vi "S2 Tool Initial.vi"(10 "process cluster":cluster{string[], i32[]}, 11 "Step Content":string[][](array[string])) -> (0 "error constant":errorcluster, 3 "S2 Initial Status":bool)   [LabVIEW 2019]
uses:
  Ctrl/StationCmdSelect.ctl
  Ctrl/Auto Inspection Station Name2.ctl
  Ctrl/Auto Inspection Data Name.ctl
  Global/Process Global.vi
  LineScan.lvclass
panel:
  in  "error in (no error)":errorcluster
  out "ToolStringOut_Init":string
  out "Initial_ChkSum":string
  in  "Numeric 3":i32
  out "Act Step":i32
  out "Numeric":dbl
  out "subarray":string[](array[string])
  out "Initial receive":string
  in  "stop":bool
  out "retry次數":string[](array[string])
  out "CurrentCmd":string
  out "Retry":i32
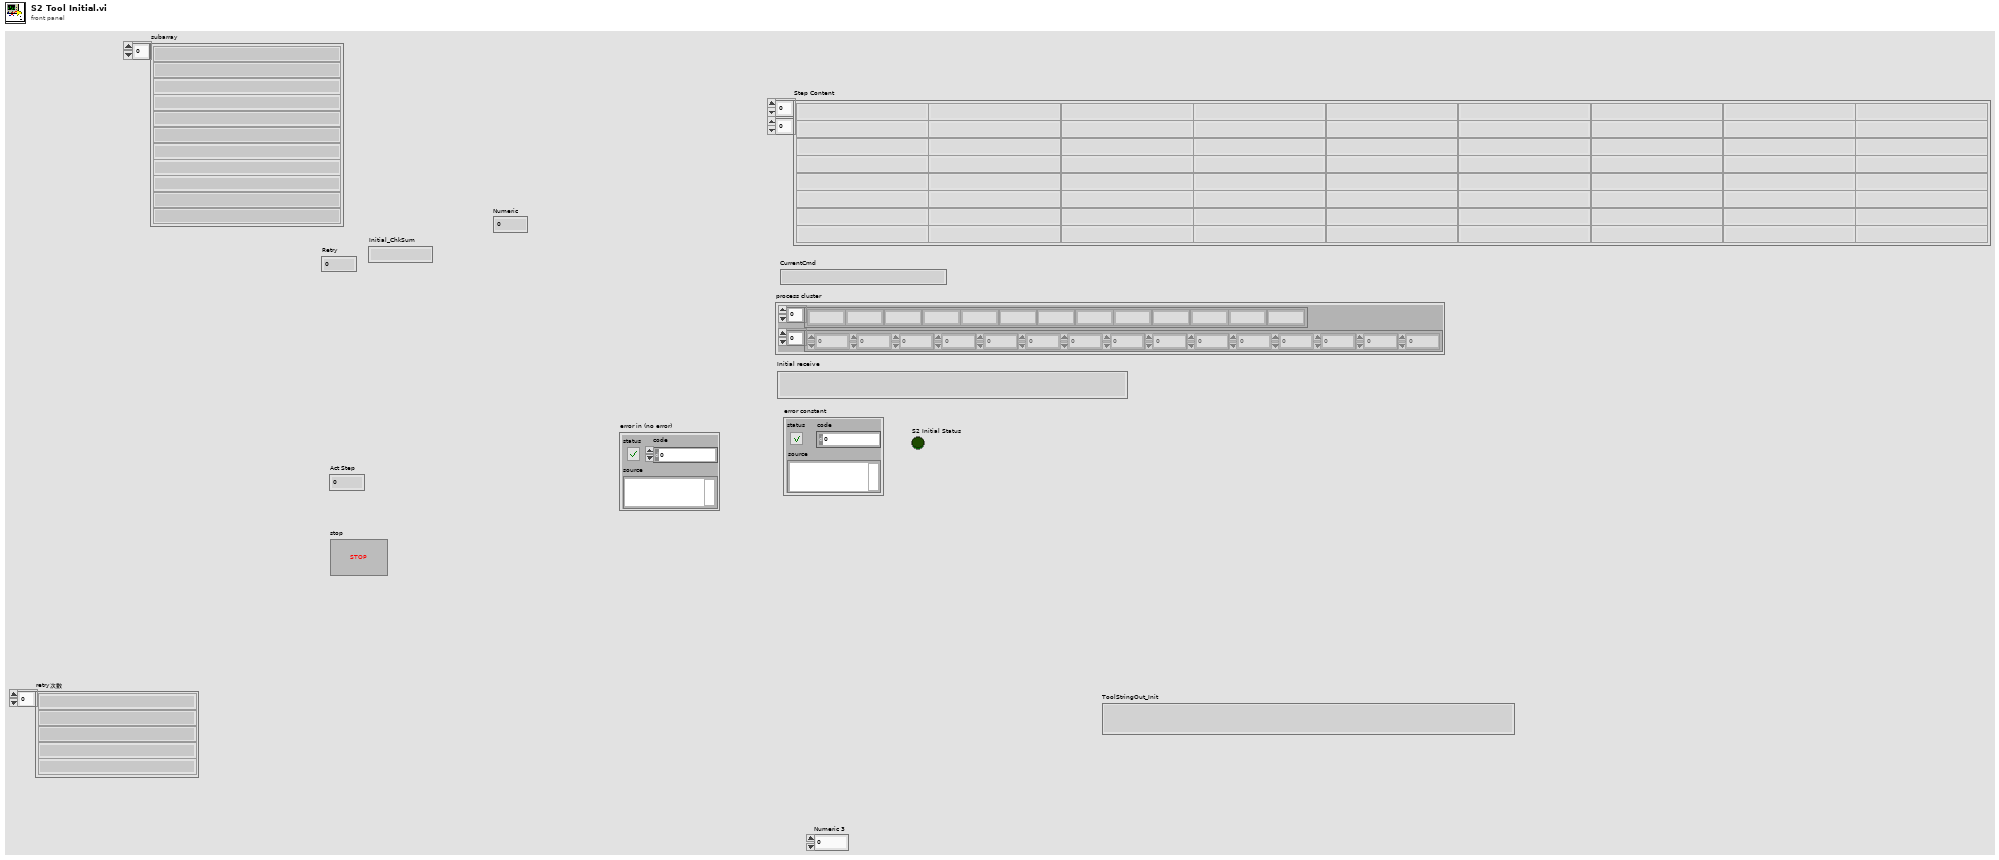
[diagram p1: front panel]
types:
  T1 = typedef "StationCmdSelect.ctl" = enum16{"Action", "Command", "Return", "DTime", "Retry"}
  T2 = typedef "Auto Inspection Data Name.ctl" = enum16{"LocalRun", "ItemSN(TimeCode)", "CurrentAction", "Error", "Data", "OKNG", "電壓值", "電壓值判斷", "電流值", "電流值判斷", "Laser1 Data", "Laser2 Data", "Laser OKNG", "StationNO"}
  T3 = typedef "Auto Inspection Station Name2.ctl" = enum16{"S1Barcode", "S2Measure", "S3Measure", "S4Measure", "S5Measure", "S11_LaserCheck", "S8_Vision AI"}
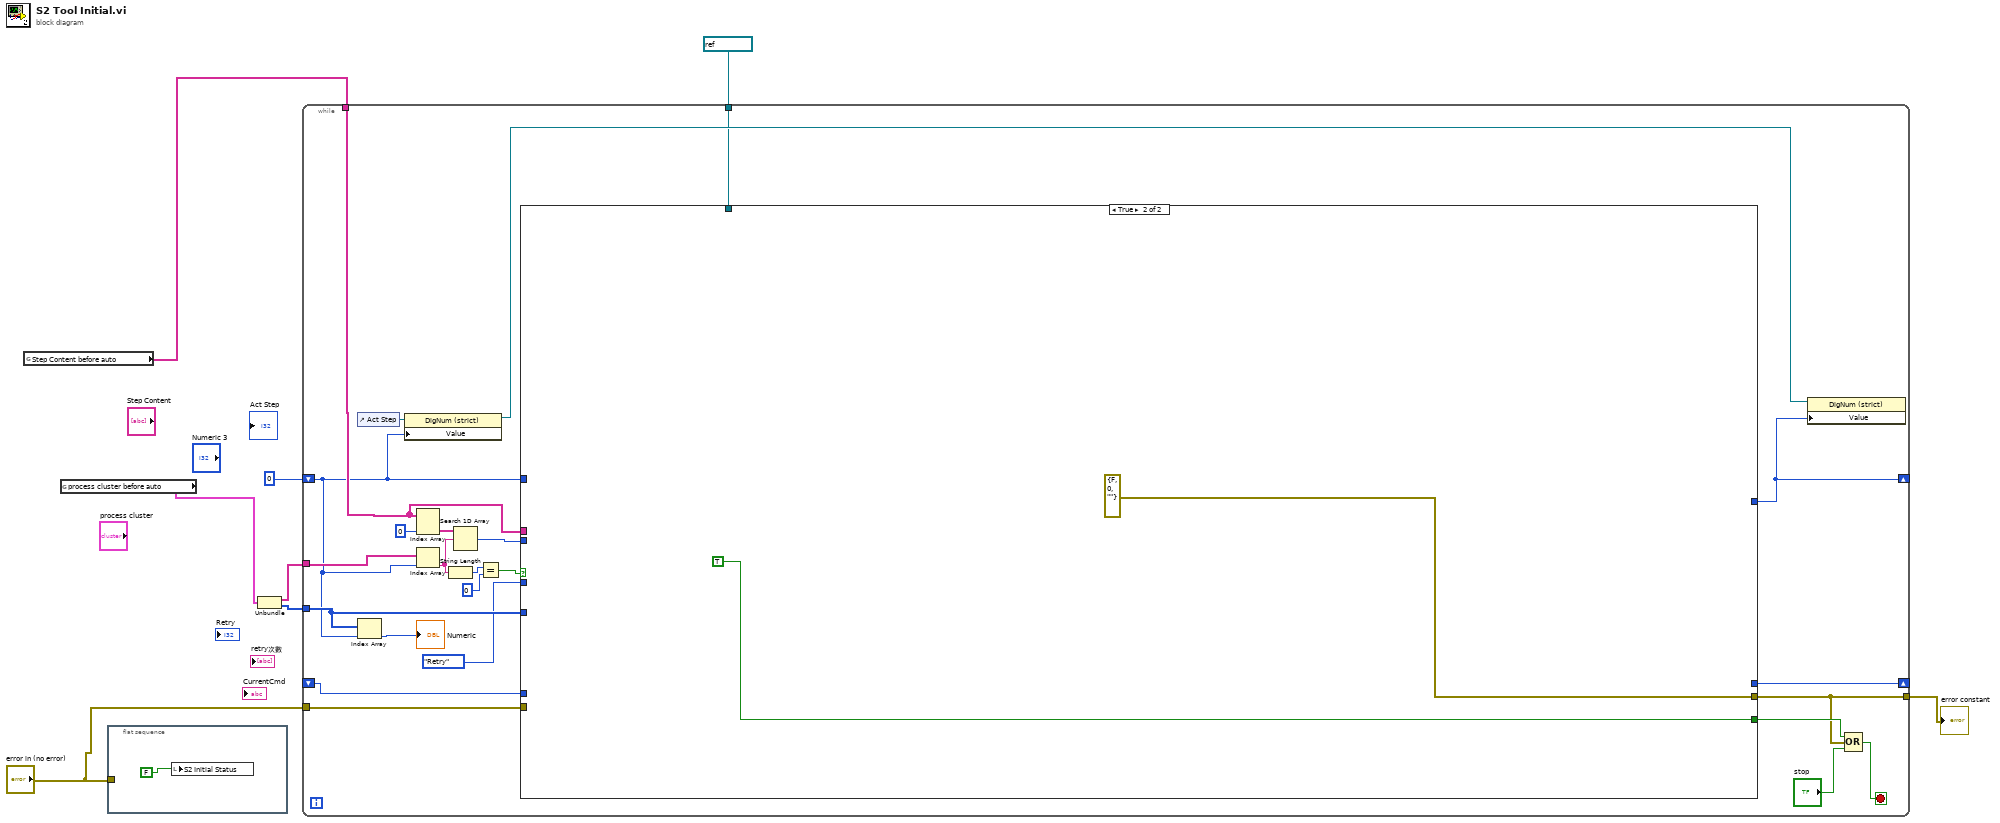
[diagram p0: block diagram]
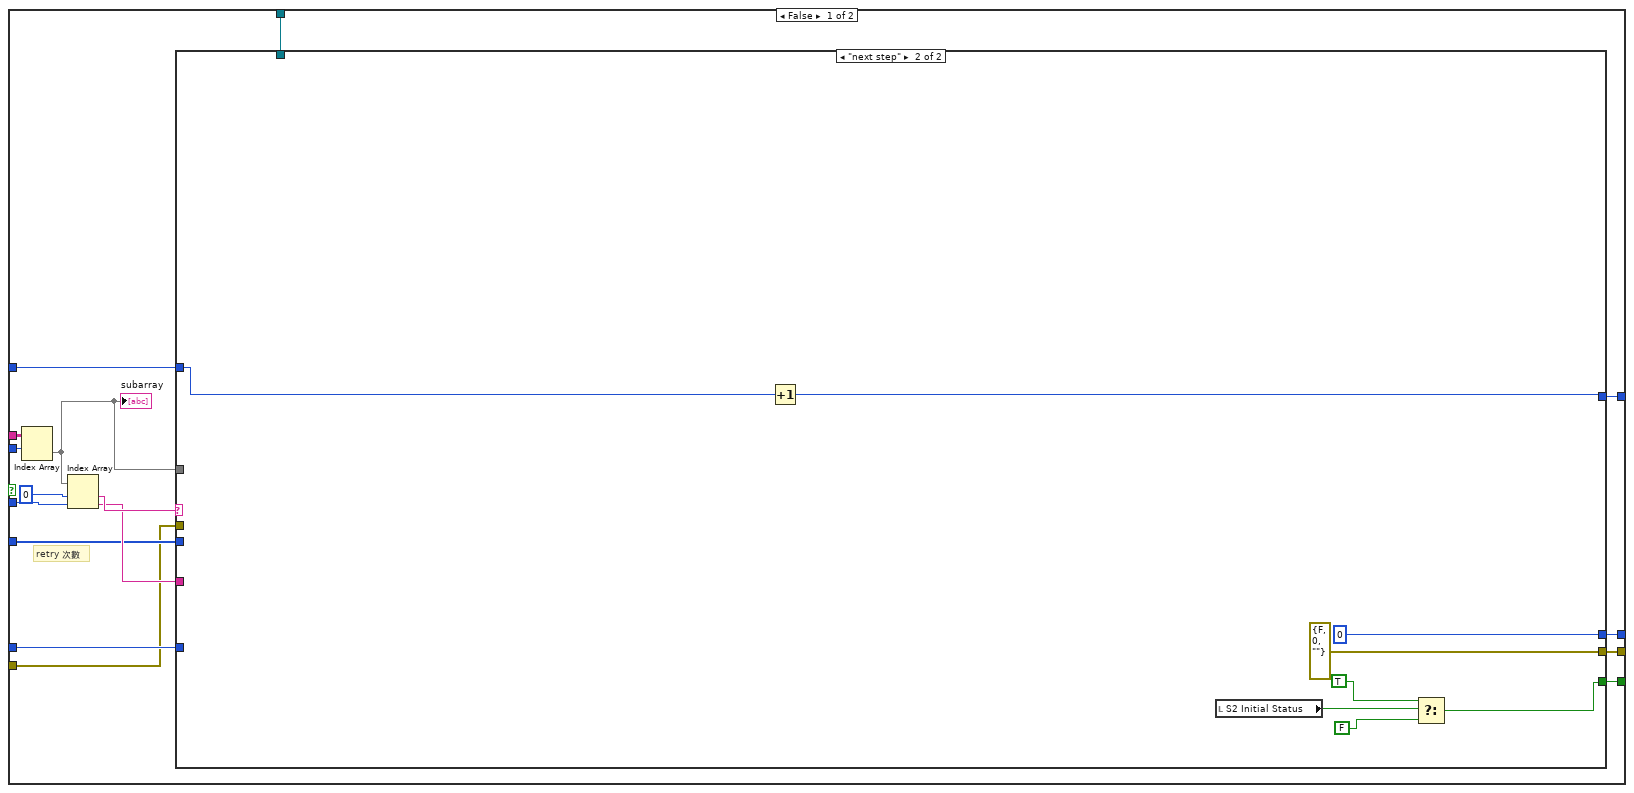
[diagram p2: hidden frame]
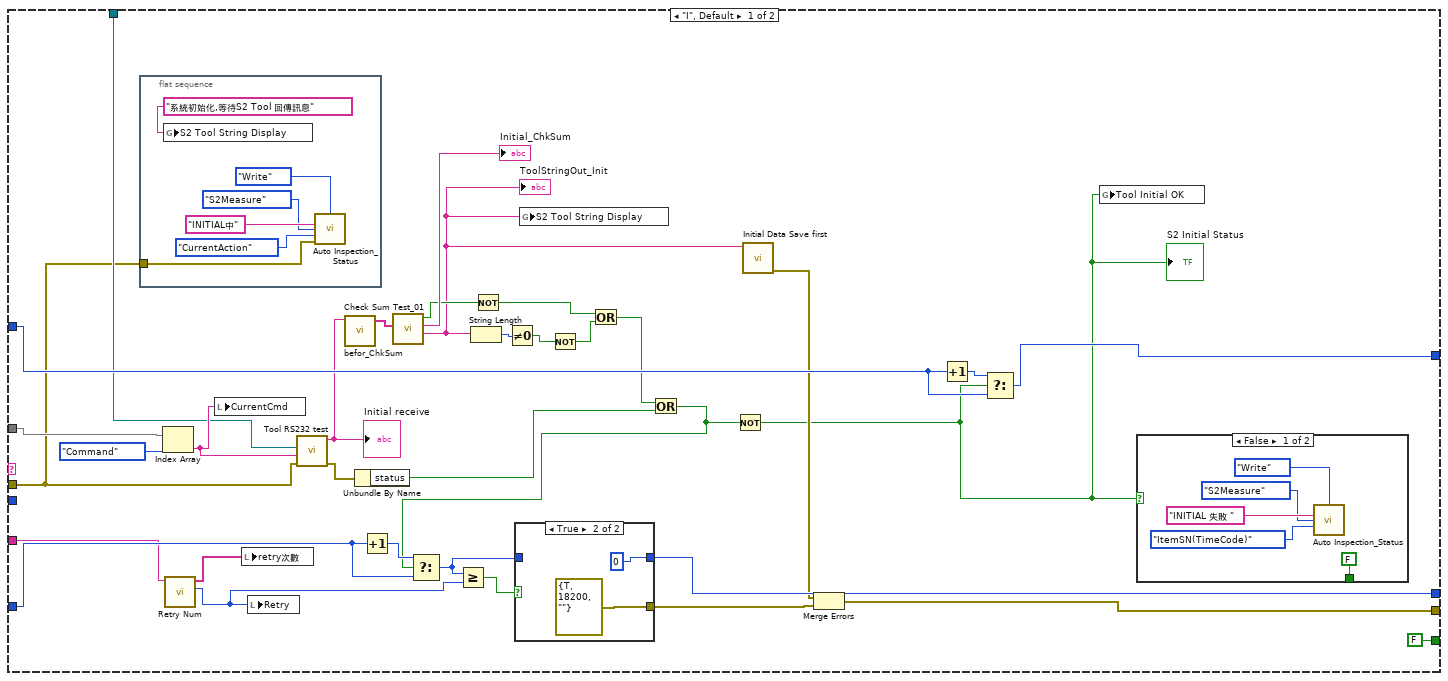
[diagram p3: hidden frame]
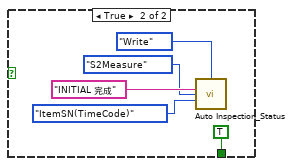
[diagram p4: hidden frame]
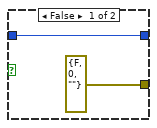
[diagram p5: hidden frame]
diagram:
  n1 = global read "Process Global.vi" "Step Content before auto"() -> (w5:string[][])
  n2 = global read "Process Global.vi" "process cluster before auto"() -> (w4:cluster{string[], i32[]})
  n3 = flat-sequence {
    tunnel: "error in (no error)" -> [_]
    frame #0 {
      n4 = local write "S2 Initial Status"(FALSE) -> ()
    }
  }
  n5 = Unbundle(w4) -> (w8:string[], w7:i32[])
  n6 = while {
    tunnel: w8 -> [w33]
    tunnel: w7 -> [w32]
    tunnel: w5 -> [w31]
    shift-right: [w15] -> _
    shift-left: _ -> [w19]
    shift-right: [w16] -> _
    shift-left: 0 ("Numeric 3") -> [w13]
    tunnel: [w12] -> w6
    tunnel: refnum<visa-resource-name> "COM1" ("VISA resource name") -> [w11]
    tunnel: "error in (no error)" -> [w10]
    stop <- w20 stop-if-true
    n7 = control-ref of="Act Step"() -> (w18:refnum<vi>)
    n8 = Index Array(array=w32, index=w13) -> (element=→"Numeric":i32)
    n9 = property class="DigNum (strict)"(reference=w18, "Value"=w13) -> (reference out=w17:refnum<vi>)  [unwired: 1 in, 1 out]
    n10 = Index Array(array=w31, index (col)=0 ("disabled index (col)")) -> (element=w29:string[])  [unwired: 1 in]
    n11 = Index Array(array=w33, index=w13) -> (element=w26:string)
    n12 = String Length(string=w26) -> (length=w25:i32)
    n13 = Search 1D Array(1D array=w29, element=w26) -> (index of element=w28:i32)  [unwired: 1 in]
    n14 = Equal?(x=w25, y=0) -> (x = y?=w23:bool)
    n15 = case shown="True" w23 {
      tunnel: w31 -> [w49 _]
      tunnel: w28 -> [w48 _]
      tunnel: w32 -> [w44 _]
      tunnel: w19 -> [w42 _]
      tunnel: StationCmdSelect."Retry" -> [w41 _]
      tunnel: [w40 errorcluster {"status"=FALSE, "code"=0, "source"=""} ("error constant")] -> w12
      tunnel: w13 -> [w39 _]
      tunnel: [w38 _] -> w16
      tunnel: [w37 _] -> w15
      tunnel: [w36 TRUE] -> w14
      tunnel: w11 -> [w35 _]
      tunnel: w10 -> [w34 _]
      frame False {
        # "retry 次數"
        n16 = Index Array(array=w49, index (row)=w48) -> (element=w43:string[])  [unwired: 1 in]
        "subarray" <- w43
        n17 = Index Array(array=w43, index #1=0 ("index"), index #2=w41) -> (element #1=w46:string, element #2=w45:string)
        n18 = case shown="\"next step\"" w46 {
          tunnel: w44 -> [_ _]
          tunnel: w45 -> [w72 _]
          tunnel: w43 -> [w74 _]
          tunnel: w42 -> [w73 _]
          tunnel: [w57 errorcluster {"status"=FALSE, "code"=0, "source"=""} ("error constant")] -> w40
          tunnel: w39 -> [w75 w111]
          tunnel: [w71 w110] -> w38
          tunnel: [w76 0] -> w37
          tunnel: [FALSE w104] -> w36
          tunnel: w34 -> [w51 _]
          tunnel: w35 -> [w56 _]
          frame "I", Default {
            n19 = flat-sequence {
              tunnel: w51 -> [w85]
              frame #0 {
                n20 = global write "Process Global.vi" "S2 Tool String Display"("系統初始化,等待S2 Tool 回傳訊息") -> ()
                n21 = call "Auto Inspection_Status.vi"("Action"=enum16{"Initial", "Write", "Read"}."Write", "DataIn"="INITIAL中", "Station"=Auto_Inspection_Station_Name2."S2Measure", "Data"=Auto_Inspection_Data_Name."CurrentAction", "error in"=w85) -> ()  [unwired: 8 in, 3 out]
              }
            }
            n22 = Index Array(array=w74, index=StationCmdSelect."Command") -> (element=w61:string)
            n23 = call "Retry Num.vi"("String"=w72) -> ("Numeric"=w81:i32, "retry次數"=w70:string[])  [unwired: 9 in]
            n24 = local write "CurrentCmd"(w61) -> ()
            n25 = local write "retry次數"(w70) -> ()
            n26 = local write "Retry"(w81) -> ()
            n27 = call "Tool RS232 test.vi"("error in (no error)"=w51, "Cmd In"=w61, "VISA resource name"=w56) -> ("error out"=w82:errorcluster, "receive string"=w52:string)  [unwired: 7 in]
            "Initial receive" <- w52
            n28 = call "befor_ChkSum.vi"("ToolString Input"=w52) -> ("Array"=w63:string[])  [unwired: 9 in, 1 out]
            n29 = Unbundle By Name(w82) -> ("status"=w69:bool)
            n30 = Increment(x=w73) -> (x+1=w83:i32)
            n31 = call "Check Sum Test_01.vi"("Array"=w63) -> ("ToolStringOut_01"=w55:string, "ChkSum"=→"Initial_ChkSum":string, "x = y?"=w59:bool)  [unwired: 8 in]
            "ToolStringOut_Init" <- w55
            n32 = String Length(string=w55) -> (length=w66:i32)
            n33 = Not(x=w59) -> (.not. x?=w64:bool)
            n34 = Not Equal To 0?(x=w66) -> (x != 0?=w67:bool)
            n35 = global write "Process Global.vi" "S2 Tool String Display"(w55) -> ()
            n36 = Not(x=w67) -> (.not. x?=w65:bool)
            n37 = Or(x=w64, y=w65) -> (x .or. y?=w60:bool)
            n38 = Or(x=w60, y=w69) -> (x .or. y?=w68:bool)
            n39 = Select(t=w83, s=w68, f=w73) -> (s? t:f=w78:i32)
            n40 = Greater Or Equal?(x=w78, y=w81) -> (x >= y?=w80:bool)
            n41 = case shown="True" w80 {
              tunnel: [errorcluster {"status"=FALSE, "code"=0, "source"=""} ("error constant") errorcluster {"status"=TRUE, "code"=18200, "source"=""} ("error constant")] -> w58
              tunnel: w78 -> [w100 _]
              tunnel: [w100 0] -> w76
              frame False {
              }
              frame True {
              }
            }
            n42 = Not(x=w68) -> (.not. x?=w50:bool)
            "S2 Initial Status" <- w50
            n43 = call "Initial Data Save first.vi"("String In"=w55) -> ("error out"=w54:errorcluster)  [unwired: 10 in]
            n44 = Merge Errors(w54, w58) -> (w57:errorcluster)
            n45 = Increment(x=w75) -> (x+1=w79:i32)
            n46 = Select(t=w79, s=w50, f=w75) -> (s? t:f=w71:i32)
            n47 = global write "Process Global.vi" "Tool Initial OK"(w50) -> ()
            n48 = case shown="False" w50 {
              tunnel: [FALSE TRUE] -> _
              frame False {
                n49 = call "Auto Inspection_Status.vi"("Action"=enum16{"Initial", "Write", "Read"}."Write", "DataIn"="INITIAL 失敗 ", "Station"=Auto_Inspection_Station_Name2."S2Measure", "Data"=Auto_Inspection_Data_Name."ItemSN(TimeCode)") -> ()  [unwired: 9 in, 3 out]
              }
              frame True {
                n50 = call "Auto Inspection_Status.vi"("Action"=enum16{"Initial", "Write", "Read"}."Write", "DataIn"="INITIAL 完成", "Station"=Auto_Inspection_Station_Name2."S2Measure", "Data"=Auto_Inspection_Data_Name."ItemSN(TimeCode)") -> ()  [unwired: 9 in, 3 out]
              }
            }
          }
          frame "next step" {
            n51 = Increment(x=w111) -> (x+1=w110:i32)
            n52 = local read "S2 Initial Status"() -> (w106:bool)
            n53 = Select(t=TRUE, s=w106, f=FALSE) -> (s? t:f=w104:bool)
          }
        }
      }
      frame True {
      }
    }
    n54 = property class="DigNum (strict)"(reference=w17, "Value"=w16) -> ()  [unwired: 1 in, 2 out]
    n55 = Compound Arithmetic op=OR(w14, w12, "stop") -> (w20:bool)
  }
  "error constant" <- w6
